vi "CreateVariantFiles.vi"   [LabVIEW 2016]
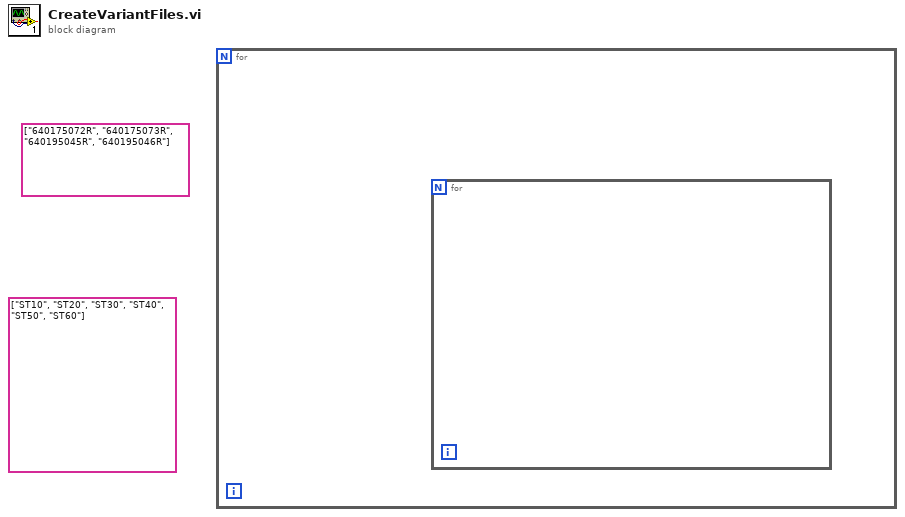
[diagram p0: block diagram]
diagram:
  (unwired) string[] ["ST10", "ST20", "ST30", "ST40", "ST50", "ST60"]
  (unwired) string[] ["640175072R", "640175073R", "640195045R", "640195046R"]
  n1 = for {
    n2 = for {
    }
  }
